vi "Write Return IED_Status Msg.vi"(10 "Return IED_Status Msg":refnum<class "Return IED_Status Msg.lvclass">, 11 "EMS Generic in":refnum<class "EMS Generic.lvclass">) -> (3 "EMS Generic out":refnum<class "EMS Generic.lvclass">)   [LabVIEW 2018, in "EMS Generic Actor.lvlib" / "EMS Generic.lvclass"]
uses:
  EMS Generic.lvclass
  EMS Generic Messages/Return IED_Status Msg/Return IED_Status Msg.lvclass
  EMS Generic.lvclass/EMS Generic.ctl
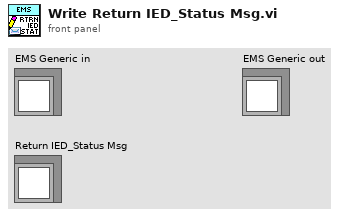
[diagram p1: front panel]
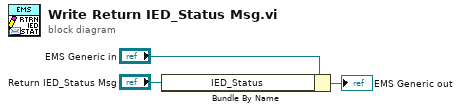
[diagram p0: block diagram]
diagram:
  n1 = Bundle By Name(cluster="EMS Generic in", "IED_Status"="Return IED_Status Msg") -> (→"EMS Generic out":refnum<class "EMS Generic.lvclass">)
